vi "even_or_odd.vi"(1 "Numeric":dbl) -> (0 "Status(Even/Odd)":string)   [LabVIEW 2020]
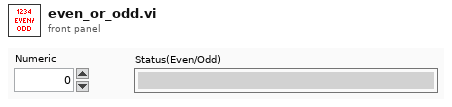
[diagram p1: front panel]
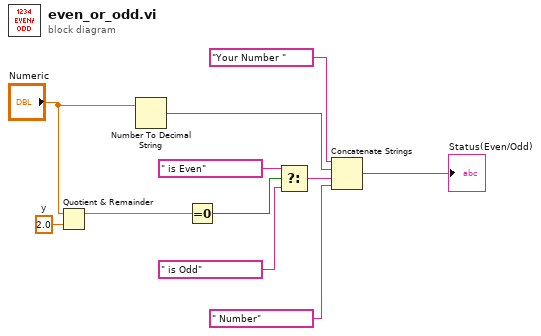
[diagram p0: block diagram]
diagram:
  w1 = 2.0  # y
  n1 = Quotient & Remainder(x="Numeric", y=w1) -> (x-y*floor(x/y)=w2:dbl)  [unwired: 1 out]
  n2 = Number To Decimal String(number="Numeric") -> (decimal integer string=w6:string)  [unwired: 1 in]
  n3 = Equal To 0?(x=w2) -> (x = 0?=w3:bool)
  n4 = Select(t=" is Even", s=w3, f=" is Odd") -> (s? t:f=w9:string)
  n5 = Concatenate Strings "Concatenate Strings"("Your Number ", w6, w9, " Number") -> (→"Status(Even/Odd)":string)
